vi "Data Window.vi"() -> ()   [LabVIEW 2019]
uses:
  SubVIs/WSData.vi
panel:
  out "Data (Raw)":dbl[](array[numeric]) format="%.2g"
  out "Data (EU)":dbl[](array[numeric]) format="%.2g"
  out "Error Out":errorcluster
  in  "Error In":errorcluster
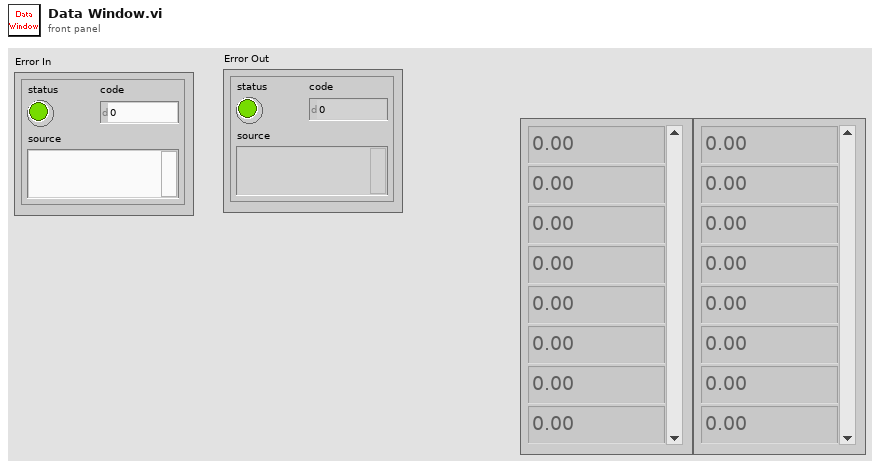
[diagram p1: front panel]
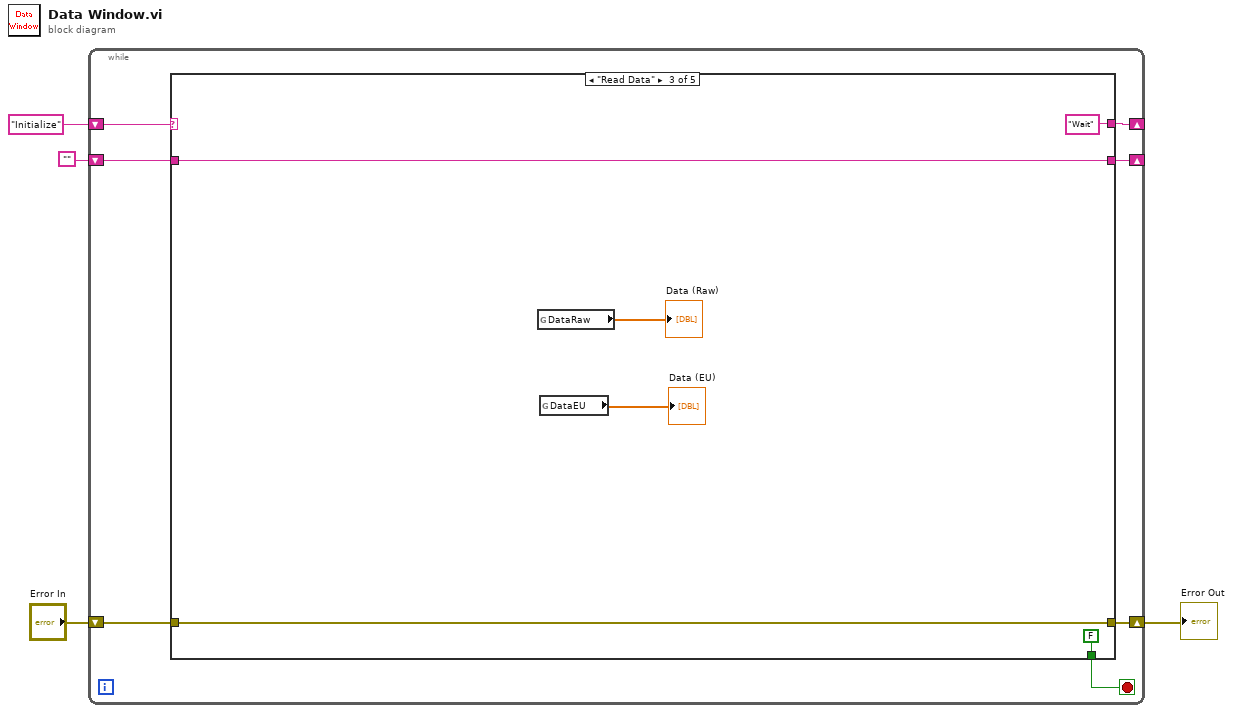
[diagram p0: block diagram]
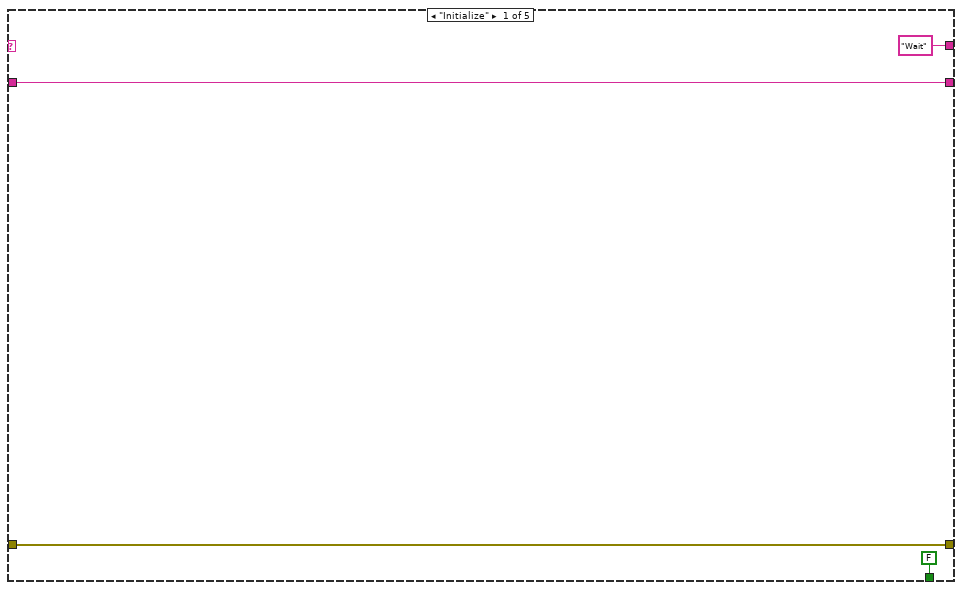
[diagram p2: hidden frame]
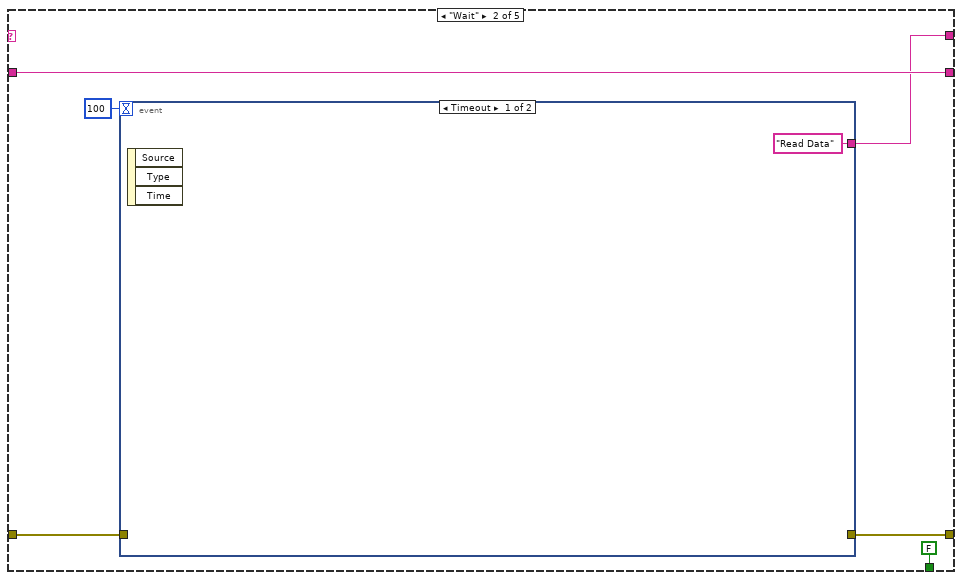
[diagram p3: hidden frame]
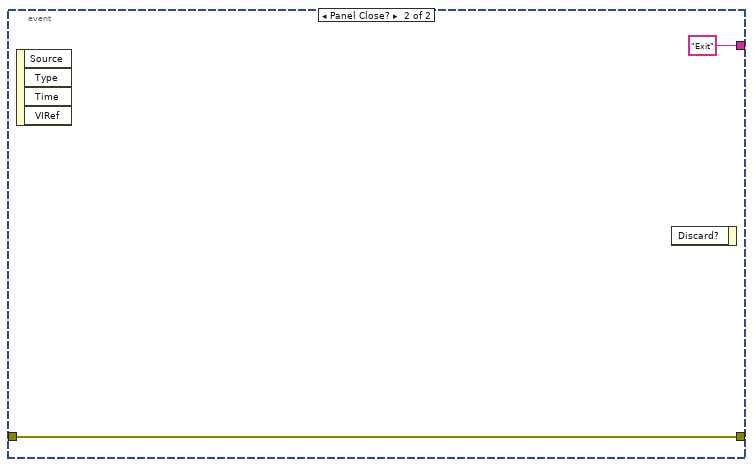
[diagram p4: hidden frame]
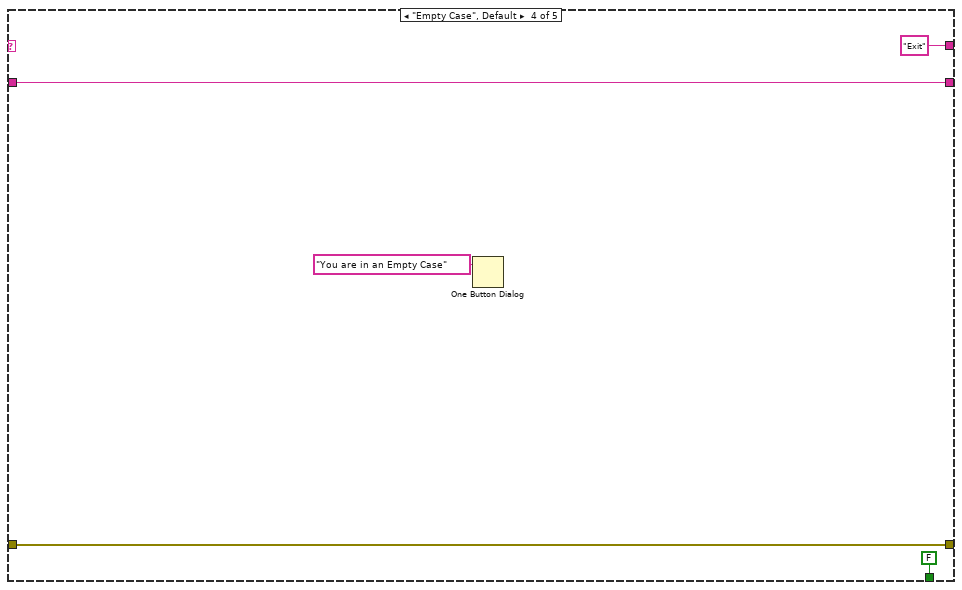
[diagram p5: hidden frame]
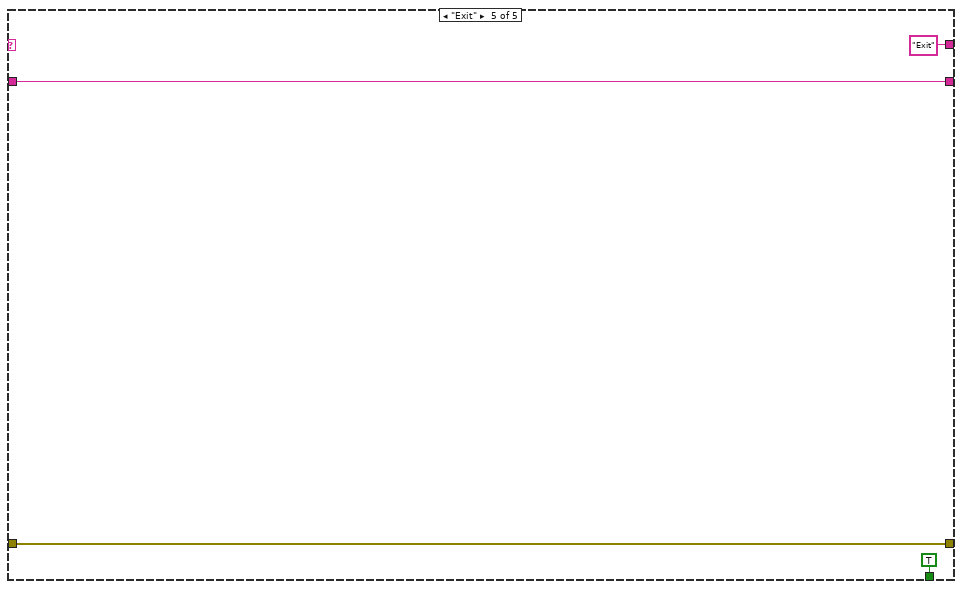
[diagram p6: hidden frame]
diagram:
  n1 = while {
    shift-right: [w7] -> _
    shift-left: "Initialize" ("key") -> [w11]
    shift-right: [w8] -> _
    shift-left: "" -> [w10]
    shift-right: [w5] -> w2
    shift-left: "Error In" -> [w9]
    stop <- w6 stop-if-true
    n2 = case shown="\"Read Data\"" w11 {
      tunnel: w10 -> [w12 w20 w27 w32 w39]
      tunnel: w9 -> [w13 w17 w28 w33 w36]
      tunnel: [w12 w20 w27 w32 w39] -> w8
      tunnel: ["Wait" ("key") w19 "Wait" ("key") "Exit" ("key") "Exit" ("key")] -> w7
      tunnel: [FALSE FALSE FALSE FALSE TRUE] -> w6
      tunnel: [w13 w16 w28 w33 w36] -> w5
      frame "Initialize" {
      }
      frame "Wait" {
        n3 = event shown="[0] Timeout" {
          selector: _ -> [_ _]
          dyn-events: _ -> [_ _]
          timeout: 100 -> [_ _]
          tunnel: ["Read Data" ("key") "Exit" ("key")] -> w19
          tunnel: w17 -> [_ w23]
          tunnel: [_ w23] -> w16
          event Timeout {
            n4 = event-data() -> ()  [unwired: 1 in, 3 out]
          }
          event Panel Close? {
            n5 = event-data() -> ()  [unwired: 1 in, 4 out]
            n6 = event-data() -> ()  [unwired: 2 in, 1 out]
          }
        }
      }
      frame "Read Data" {
        n7 = global read "WSData.vi" "DataRaw"() -> (→"Data (Raw)":dbl[])
        n8 = global read "WSData.vi" "DataEU"() -> (→"Data (EU)":dbl[])
      }
      frame "Empty Case", Default {
        n9 = One Button Dialog(message="You are in an Empty Case") -> ()  [unwired: 1 in, 1 out]
      }
      frame "Exit" {
      }
    }
  }
  "Error Out" <- w2
